vi "Shutdown Helper Loop.vi"(11 "XY Stage Process in":refnum<class "XY Stage Process.lvclass">) -> ()   [LabVIEW 2022 SP3, in "XY Stage Process.lvlib" / "XY Stage Process.lvclass"]
uses:
  XY Stage Process.lvclass
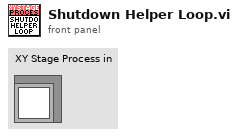
[diagram p1: front panel]
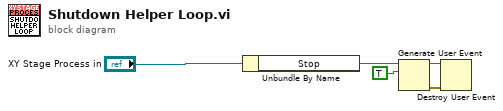
[diagram p0: block diagram]
diagram:
  n1 = Unbundle By Name("XY Stage Process in") -> ("Stop"=w2:refnum<user-event>)
  n2 = Generate User Event(user event=w2, event data cluster=TRUE) -> (user event out=w5:refnum<user-event>, error out=w4:errorcluster)  [unwired: 2 in]
  n3 = Destroy User Event(user event=w5, error in=w4) -> ()  [unwired: 1 out]
